vi "Upgrade Package.vi"(8 "error in (no error)":errorcluster, 10 "Version String (Latest)":string, 11 "Package in":refnum<class "Package.lvclass">) -> (0 "error out":errorcluster, 3 "Package out":refnum<class "Package.lvclass">)   [LabVIEW 2020, in "neg-pkg.lvlib" / "Package.lvclass"]
uses:
  Package.lvclass
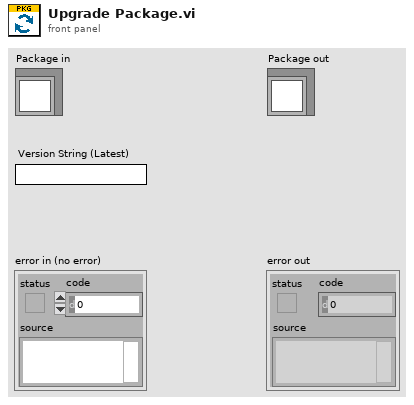
[diagram p1: front panel]
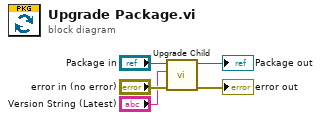
[diagram p0: block diagram]
diagram:
  n1 = call-dynamic "Upgrade Child.vi"("error in (no error)"="error in (no error)", "Version String (Latest)"="Version String (Latest)", "Package in"="Package in") -> ("error out"=→"error out":errorcluster, "Package out"=→"Package out":refnum<class "Package.lvclass">)  [unwired: 7 in]
